vi "Calc Cmd Chans.vi"(8 "error in (no error)":errorcluster, 11 "Tare Calc in":refnum<class "Tare Calc.lvclass">) -> (0 "error out":errorcluster, 1 "Numeric Cmd Chans":string[](array[string]), 2 "Digital Cmd Chans":string[](array[string]), 3 "Tare Calc out":refnum<class "Tare Calc.lvclass">)   [LabVIEW 2020, in "VolatusCalcs.lvlib" / "Tare Calc.lvclass"]
uses:
  Tare Calc.lvclass
  Tare Calc.lvclass/Tare Calc.ctl
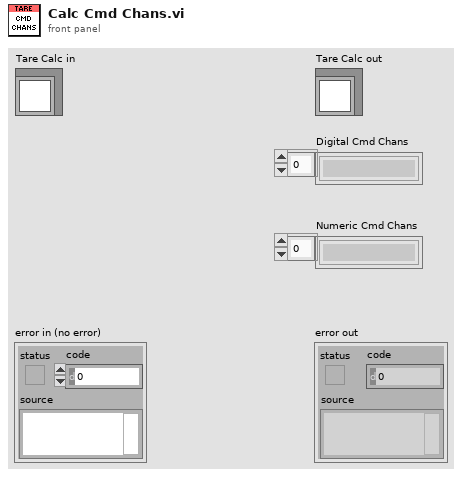
[diagram p1: front panel]
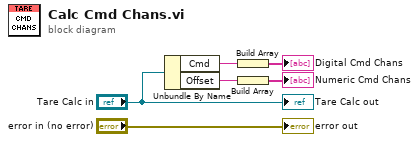
[diagram p0: block diagram]
diagram:
  n1 = Unbundle By Name("Tare Calc in") -> ("Cmd"=w4:string, "Offset"=w3:string)
  n2 = Build Array(w4) -> (→"Digital Cmd Chans":string[])
  n3 = Build Array(w3) -> (→"Numeric Cmd Chans":string[])
  "error out" <- "error in (no error)"
  "Tare Calc out" <- "Tare Calc in"
